vi "REPORT.Rate scan ADD.vi"(9 "Vasic":i32, 10 "Config Test IN":T1={"Config HW"={"VISA Rigol DP832"="USB0::0x1AB1::0x0E11::DP8C191500901::INSTR", "Config Rigol DP832"=[{"Channel"=0, "V Limit"=5.5, "I Limit"=0.5, "V Out"=5.0}, {"Channel"=1, "V Limit"=5.5, "I Limit"=0.8, "V Out"=5.0}, {"Channel"=2, "V Limit"=5.5, "I Limit"=0.2, "V Out"=0.0}], "CTA Test#"="CTA013 A", "FT_Handle"=432921256, "Espera acceso FT"=10, "VISA Tek MDO3104"="Rigol_DP832", "VISA Key 81160A"="Rigol_DP832"}, "Config Test"=[{"Vasic"=2.8, "Global Reset"=FALSE, "Test Register?"=FALSE, "Test ADC?"=FALSE, "Test ADC"={"Repeats ADC"=100, "Max Desviation"=0.1}, "Limits ADC"={"Low"=[1.9, 1.3, 0.65, 0.0, 1.6, 1.4, 1.4, 0.9, 2.1, 0.85, 1.9], "High"=[2.1, 1.5, 0.85, 0.1, 1.4, 1.2, 1.2, 0.7, 1.9, 0.65, 1.7]}, "Test Max PN Min NP?"=FALSE, "Limits Max PN Min NP"={"Max P Upper"=2.177000045776367, "Min P Upper"=1.474, "Max N Upper"=1.475, "Min N Upper"=0.818, "Max P Lower"=1.888, "Min P Lower "=1.321, "Max N Lower"=1.322, "Min N Lower"=0.73}, "Test Rate Scan?"=FALSE, "Vin Rate Scan"=[], "Limits Rate Scan"={"High"=[0.15, 0.242, 0.331, 0.425, 0.512, 0.6, 0.688, 0.774, 0.847, 0.91], "Low"=[0.021, 0.11, 0.189, 0.27, 0.347, 0.421, 0.487, 0.551, 0.601, 0.635]}, "Test Rate Scan Adders?"=FALSE, "Vin Rate Adders"=[], "Limits Rate Scan adders"={"High"=[], "Low"=[]}, "Test offset analog?"=FALSE, "Lim Offset Analog"={"Max Analog"=0.05, "Min Analog"=-0.05}, "Test offset digital?"=FALSE, "Lim offset Dig"={"Max Dig"=0.05}, "Vasic real f.a."=2.8, "IBIAS"=FALSE, "VALUE IBIAS"=63}, {"Vasic"=2.8, "Global Reset"=FALSE, "Test Register?"=FALSE, "Test ADC?"=FALSE, "Test ADC"={"Repeats ADC"=100, "Max Desviation"=0.1}, "Limits ADC"={"Low"=[1.9, 1.3, 0.65, 0.0, 1.6, 1.4, 1.4, 0.9, 2.1, 0.85, 1.9], "High"=[2.1, 1.5, 0.85, 0.1, 1.4, 1.2, 1.2, 0.7, 1.9, 0.65, 1.7]}, "Test Max PN Min NP?"=FALSE, "Limits Max PN Min NP"={"Max P Upper"=2.177000045776367, "Min P Upper"=1.474, "Max N Upper"=1.475, "Min N Upper"=0.818, "Max P Lower"=1.888, "Min P Lower "=1.321, "Max N Lower"=1.322, "Min N Lower"=0.73}, "Test Rate Scan?"=FALSE, "Vin Rate Scan"=[], "Limits Rate Scan"={"High"=[0.15, 0.242, 0.331, 0.425, 0.512, 0.6, 0.688, 0.774, 0.847, 0.91], "Low"=[0.021, 0.11, 0.189, 0.27, 0.347, 0.421, 0.487, 0.551, 0.601, 0.635]}, "Test Rate Scan Adders?"=FALSE, "Vin Rate Adders"=[], "Limits Rate Scan adders"={"High"=[], "Low"=[]}, "Test offset analog?"=FALSE, "Lim Offset Analog"={"Max Analog"=0.05, "Min Analog"=-0.05}, "Test offset digital?"=FALSE, "Lim offset Dig"={"Max Dig"=0.05}, "Vasic real f.a."=2.8, "IBIAS"=FALSE, "VALUE IBIAS"=63}, {"Vasic"=2.8, "Global Reset"=FALSE, "Test Register?"=FALSE, "Test ADC?"=FALSE, "Test ADC"={"Repeats ADC"=100, "Max Desviation"=0.1}, "Limits ADC"={"Low"=[1.9, 1.3, 0.65, 0.0, 1.6, 1.4, 1.4, 0.9, 2.1, 0.85, 1.9], "High"=[2.1, 1.5, 0.85, 0.1, 1.4, 1.2, 1.2, 0.7, 1.9, 0.65, 1.7]}, "Test Max PN Min NP?"=FALSE, "Limits Max PN Min NP"={"Max P Upper"=2.177000045776367, "Min P Upper"=1.474, "Max N Upper"=1.475, "Min N Upper"=0.818, "Max P Lower"=1.888, "Min P Lower "=1.321, "Max N Lower"=1.322, "Min N Lower"=0.73}, "Test Rate Scan?"=FALSE, "Vin Rate Scan"=[], "Limits Rate Scan"={"High"=[0.15, 0.242, 0.331, 0.425, 0.512, 0.6, 0.688, 0.774, 0.847, 0.91], "Low"=[0.021, 0.11, 0.189, 0.27, 0.347, 0.421, 0.487, 0.551, 0.601, 0.635]}, "Test Rate Scan Adders?"=FALSE, "Vin Rate Adders"=[], "Limits Rate Scan adders"={"High"=[], "Low"=[]}, "Test offset analog?"=FALSE, "Lim Offset Analog"={"Max Analog"=0.05, "Min Analog"=-0.05}, "Test offset digital?"=FALSE, "Lim offset Dig"={"Max Dig"=0.05}, "Vasic real f.a."=2.8, "IBIAS"=FALSE, "VALUE IBIAS"=63}, {"Vasic"=2.8, "Global Reset"=FALSE, "Test Register?"=FALSE, "Test ADC?"=FALSE, "Test ADC"={"Repeats ADC"=100, "Max Desviation"=0.1}, "Limits ADC"={"Low"=[1.9, 1.3, 0.65, 0.0, 1.6, 1.4, 1.4, 0.9, 2.1, 0.85, 1.9], "High"=[2.1, 1.5, 0.85, 0.1, 1.4, 1.2, 1.2, 0.7, 1.9, 0.65, 1.7]}, "Test Max PN Min NP?"=FALSE, "Limits Max PN Min NP"={"Max P Upper"=2.177000045776367, "Min P Upper"=1.474, "Max N Upper"=1.475, "Min N Upper"=0.818, "Max P Lower"=1.888, "Min P Lower "=1.321, "Max N Lower"=1.322, "Min N Lower"=0.73}, "Test Rate Scan?"=FALSE, "Vin Rate Scan"=[], "Limits Rate Scan"={"High"=[0.15, 0.242, 0.331, 0.425, 0.512, 0.6, 0.688, 0.774, 0.847, 0.91], "Low"=[0.021, 0.11, 0.189, 0.27, 0.347, 0.421, 0.487, 0.551, 0.601, 0.635]}, "Test Rate Scan Adders?"=FALSE, "Vin Rate Adders"=[], "Limits Rate Scan adders"={"High"=[], "Low"=[]}, "Test offset analog?"=FALSE, "Lim Offset Analog"={"Max Analog"=0.05, "Min Analog"=-0.05}, "Test offset digital?"=FALSE, "Lim offset Dig"={"Max Dig"=0.05}, "Vasic real f.a."=2.8, "IBIAS"=FALSE, "VALUE IBIAS"=63}], "Result"=[{"Vasic Volt"=0, "Test Registros"={"Default Register OK"=TRUE, "Pattern Default"=[6826, 18761, 18761, 18761, 30576, 383, 13312], "Read Default"=[6826, 18761, 18761, 18761, 30576, 383, 13312], "W/R Register OK"=TRUE, "Pattern W/R"=[58709, 46774, 46774, 46774, 34959, 65152, 52223], "Read W/R"=[58709, 46774, 46774, 46774, 34959, 65152, 52223]}, "Test Dacs"={"Desviacion OK"=TRUE, "Means"=[1.9590537240537238, 1.3874725274725273, 0.7671367521367521, 0.020757020757020753, 1.5494139194139194, 1.303919413919414, 1.2742918192918191, 1.2090720390720389, 0.7778327228327229, 2.0368192918192918, 1.8345909645909646], "Deviations"=[0.00042735042735042583, 0.0003965050749137904, 0.00033891407793921574, 3.486925384749193e-18, 0.000366300366300365, 0.0009361009361009328, 0.0010387212621211883, 0.00037241598701881083, 0.0002311318008058711, 0.00043985325898711266, 0.00036630036630038717], "Desviations OK"=[], "Means OK"=[], "Graph Histogram"=[]}, "Test Max-Min PN"={"Max P Mini N OK"=TRUE, "PTHT Max P Min N"=[1.956043956043956, 1.9566544566544566, 1.9566544566544566, 2.034188034188034, 2.0354090354090353, 2.0347985347985347], "PTHT Max P Min N OK"=[TRUE, TRUE, TRUE, TRUE, TRUE, TRUE], "NTHT Max P Min N"=[0.7673992673992674, 0.7673992673992674, 0.7680097680097681, 0.778998778998779, 0.7796092796092796, 0.7796092796092796], "NTHT Max P Min N OK"=[TRUE, TRUE, TRUE, TRUE, TRUE, TRUE], "Min P Max N OK"=TRUE, "PTHT Max N Min P"=[1.387057387057387, 1.387057387057387, 1.387057387057387, 1.4059829059829059, 1.4078144078144077, 1.407203907203907], "PTHT Max N Min P OK"=[TRUE, TRUE, TRUE, TRUE, TRUE, TRUE], "NTHT Max N Min P"=[1.3858363858363858, 1.3846153846153846, 1.3852258852258852, 1.404151404151404, 1.4047619047619047, 1.404151404151404], "NTHT Max N Min P OK"=[TRUE, TRUE, TRUE, TRUE, TRUE, TRUE], "Ref"=[{"DAC THx"=0}, {"DAC THx"=1}, {"DAC THx"=2}, {"DAC THx"=3}, {"DAC THx"=4}, {"DAC THx"=5}]}, "Test Rate Scan"={"Rate Scan OK"=FALSE, "DAC TH0,TH1,TH2"=[], "Volt HLTH"=[], "Rate HLTH OK"=[], "DAC TH3,TH4,TH5"=[], "Volt LLTH"=[], "Rate LLTH 2 OK"=[], "Scaler 0"=[], "Ref"=[], "OFFSET HLTH"=[], "OFFSET LLTH"=[], "Real Voltage"=[]}, "Test Rate Scan adders"={"Rate Scan Adders OK"=FALSE, "DAC TH0,TH1,TH2"=[[[142, 132, 122], [146, 136, 124], [146, 136, 126], [206, 196, 184], [210, 202, 188], [210, 198, 186], [270, 260, 246], [270, 262, 248], [268, 258, 244]], [[248, 238, 222], [250, 242, 226], [250, 242, 228], [358, 348, 330], [360, 352, 334], [358, 350, 334], [460, 452, 434], [462, 454, 438], [458, 450, 434]]], "Volt HLTH"=[[[0.16544566544566552, 0.1562881562881564, 0.14285714285714302], [0.16971916971916978, 0.16117216117216127, 0.14713064713064727], [0.16971916971916978, 0.16117216117216127, 0.14774114774114788], [0.23992673992673996, 0.23015873015873023, 0.21611721611721624], [0.24420024420024422, 0.2362637362637363, 0.2210012210012211], [0.24420024420024422, 0.23137973137973145, 0.21733821733821745], [0.313797313797314, 0.30463980463980467, 0.286935286935287], [0.313797313797314, 0.3058608058608059, 0.2905982905982907], [0.3125763125763128, 0.300976800976801, 0.2851037851037852]], [[0.28937728937728946, 0.2771672771672773, 0.2588522588522588], [0.2905982905982907, 0.28205128205128216, 0.2637362637362637], [0.2905982905982907, 0.28205128205128216, 0.26678876678876673], [0.4157509157509156, 0.4059829059829059, 0.384004884004884], [0.41941391941391926, 0.41086691086691074, 0.38888888888888884], [0.4157509157509156, 0.4072039072039071, 0.38827838827838823], [0.5354090354090353, 0.5268620268620268, 0.5048840048840049], [0.5366300366300365, 0.5274725274725274, 0.5091575091575091], [0.5317460317460316, 0.5225885225885225, 0.5042735042735043]]], "Add HLTH OK"=[], "DAC TH3,TH4,TH5"=[], "Volt LLTH"=[[[134.0, 122.0, 114.0], [136.0, 126.0, 118.0], [136.0, 126.0, 118.0], [192.0, 182.0, 174.0], [194.0, 186.0, 178.0], [194.0, 186.0, 176.0], [250.0, 242.0, 234.0], [254.0, 244.0, 234.0], [250.0, 240.0, 230.0]], [[230.0, 220.0, 212.0], [234.0, 224.0, 214.0], [234.0, 224.0, 214.0], [338.0, 326.0, 316.0], [338.0, 330.0, 320.0], [338.0, 328.0, 318.0], [436.0, 424.0, 416.0], [438.0, 426.0, 416.0], [434.0, 422.0, 414.0]]], "Add LLTH 2 OK"=[], "Scaler 0"=[[[1, 1, 1], [1, 1, 1], [1, 1, 1], [0, 0, 0], [0, 0, 0], [0, 0, 0], [0, 0, 0], [0, 0, 0], [0, 0, 0]], [[1, 1, 1], [1, 1, 1], [1, 1, 1], [0, 1, 1], [0, 1, 1], [0, 1, 1], [0, 0, 0], [0, 0, 0], [0, 0, 0]]], "Ref"=[], "OFFSET HLTH"=[], "OFFSET LLTH"=[], "Real Voltage"=[]}, "Test Offset Analog"={"Offset Analog OK"=FALSE, "V ADDOUT"=[], "Offset OK"=[], "Ref"=[]}, "Test Offset Digital"={"Offset Digital OK"=FALSE, "SCALER 1 START"=[], "SCALER 1 STOP"=[], "THX START"=[], "THX STOP"=[], "VHLTH START"=[], "VHLTH STOP"=[], "Index 1 Start"=[], "index 1 Stop"=[], "SCALER 2 START"=[], "SCALER 2 STOP"=[], "THX+3 START"=[], "THX+3 STOP"=[], "VLLTH START"=[], "VLLTH STOP"=[], "Index 2 Start"=[], "index 2 Stop"=[], "Dig HLTH OK"=[], "Dig LLTH 2 OK"=[], "Ref"=[]}, "info hardware"={"Iout V1"=0.0, "Iout V2"=0.0, "Iout V3"=0.0, "Vout V1"=0.0, "Vout V2"=0.0, "Vout V3"=0.0, "Temp"=0.0}, "Test Offset Analog add"={"Offset Analog add OK"=FALSE, "V ADDOUT add"=[], "Offset add OK"=[], "Ref add"=[]}, "info temp"={"T Asic Registers"=0.0, "T Board Test. ADC"=0.0, "T Asic Max Min N P"=0.0, "T Adc count"=0.0, "T Asic Digital Offset"=0.0, "T Asic Analog Offset"=0.0, "T Asic Analog add"=0.0, "T Asic Rate Scan"=0.0, "T Asic Rate Scan Adders"=0.0, "T Final"=0.0}}, {"Vasic Volt"=0, "Test Registros"={"Default Register OK"=TRUE, "Pattern Default"=[6826, 18761, 18761, 18761, 30576, 383, 13312], "Read Default"=[6826, 18761, 18761, 18761, 30576, 383, 13312], "W/R Register OK"=TRUE, "Pattern W/R"=[58709, 46774, 46774, 46774, 34959, 65152, 52223], "Read W/R"=[58709, 46774, 46774, 46774, 34959, 65152, 52223]}, "Test Dacs"={"Desviacion OK"=TRUE, "Means"=[1.9590537240537238, 1.3874725274725273, 0.7671367521367521, 0.020757020757020753, 1.5494139194139194, 1.303919413919414, 1.2742918192918191, 1.2090720390720389, 0.7778327228327229, 2.0368192918192918, 1.8345909645909646], "Deviations"=[0.00042735042735042583, 0.0003965050749137904, 0.00033891407793921574, 3.486925384749193e-18, 0.000366300366300365, 0.0009361009361009328, 0.0010387212621211883, 0.00037241598701881083, 0.0002311318008058711, 0.00043985325898711266, 0.00036630036630038717], "Desviations OK"=[], "Means OK"=[], "Graph Histogram"=[]}, "Test Max-Min PN"={"Max P Mini N OK"=TRUE, "PTHT Max P Min N"=[1.956043956043956, 1.9566544566544566, 1.9566544566544566, 2.034188034188034, 2.0354090354090353, 2.0347985347985347], "PTHT Max P Min N OK"=[TRUE, TRUE, TRUE, TRUE, TRUE, TRUE], "NTHT Max P Min N"=[0.7673992673992674, 0.7673992673992674, 0.7680097680097681, 0.778998778998779, 0.7796092796092796, 0.7796092796092796], "NTHT Max P Min N OK"=[TRUE, TRUE, TRUE, TRUE, TRUE, TRUE], "Min P Max N OK"=TRUE, "PTHT Max N Min P"=[1.387057387057387, 1.387057387057387, 1.387057387057387, 1.4059829059829059, 1.4078144078144077, 1.407203907203907], "PTHT Max N Min P OK"=[TRUE, TRUE, TRUE, TRUE, TRUE, TRUE], "NTHT Max N Min P"=[1.3858363858363858, 1.3846153846153846, 1.3852258852258852, 1.404151404151404, 1.4047619047619047, 1.404151404151404], "NTHT Max N Min P OK"=[TRUE, TRUE, TRUE, TRUE, TRUE, TRUE], "Ref"=[{"DAC THx"=0}, {"DAC THx"=1}, {"DAC THx"=2}, {"DAC THx"=3}, {"DAC THx"=4}, {"DAC THx"=5}]}, "Test Rate Scan"={"Rate Scan OK"=FALSE, "DAC TH0,TH1,TH2"=[], "Volt HLTH"=[], "Rate HLTH OK"=[], "DAC TH3,TH4,TH5"=[], "Volt LLTH"=[], "Rate LLTH 2 OK"=[], "Scaler 0"=[], "Ref"=[], "OFFSET HLTH"=[], "OFFSET LLTH"=[], "Real Voltage"=[]}, "Test Rate Scan adders"={"Rate Scan Adders OK"=FALSE, "DAC TH0,TH1,TH2"=[], "Volt HLTH"=[], "Add HLTH OK"=[], "DAC TH3,TH4,TH5"=[], "Volt LLTH"=[], "Add LLTH 2 OK"=[], "Scaler 0"=[], "Ref"=[], "OFFSET HLTH"=[], "OFFSET LLTH"=[], "Real Voltage"=[]}, "Test Offset Analog"={"Offset Analog OK"=FALSE, "V ADDOUT"=[], "Offset OK"=[], "Ref"=[]}, "Test Offset Digital"={"Offset Digital OK"=FALSE, "SCALER 1 START"=[], "SCALER 1 STOP"=[], "THX START"=[], "THX STOP"=[], "VHLTH START"=[], "VHLTH STOP"=[], "Index 1 Start"=[], "index 1 Stop"=[], "SCALER 2 START"=[], "SCALER 2 STOP"=[], "THX+3 START"=[], "THX+3 STOP"=[], "VLLTH START"=[], "VLLTH STOP"=[], "Index 2 Start"=[], "index 2 Stop"=[], "Dig HLTH OK"=[], "Dig LLTH 2 OK"=[], "Ref"=[]}, "info hardware"={"Iout V1"=0.0, "Iout V2"=0.0, "Iout V3"=0.0, "Vout V1"=0.0, "Vout V2"=0.0, "Vout V3"=0.0, "Temp"=0.0}, "Test Offset Analog add"={"Offset Analog add OK"=FALSE, "V ADDOUT add"=[], "Offset add OK"=[], "Ref add"=[]}, "info temp"={"T Asic Registers"=0.0, "T Board Test. ADC"=0.0, "T Asic Max Min N P"=0.0, "T Adc count"=0.0, "T Asic Digital Offset"=0.0, "T Asic Analog Offset"=0.0, "T Asic Analog add"=0.0, "T Asic Rate Scan"=0.0, "T Asic Rate Scan Adders"=0.0, "T Final"=0.0}}, {"Vasic Volt"=0, "Test Registros"={"Default Register OK"=TRUE, "Pattern Default"=[6826, 18761, 18761, 18761, 30576, 383, 13312], "Read Default"=[6826, 18761, 18761, 18761, 30576, 383, 13312], "W/R Register OK"=TRUE, "Pattern W/R"=[58709, 46774, 46774, 46774, 34959, 65152, 52223], "Read W/R"=[58709, 46774, 46774, 46774, 34959, 65152, 52223]}, "Test Dacs"={"Desviacion OK"=TRUE, "Means"=[1.9590537240537238, 1.3874725274725273, 0.7671367521367521, 0.020757020757020753, 1.5494139194139194, 1.303919413919414, 1.2742918192918191, 1.2090720390720389, 0.7778327228327229, 2.0368192918192918, 1.8345909645909646], "Deviations"=[0.00042735042735042583, 0.0003965050749137904, 0.00033891407793921574, 3.486925384749193e-18, 0.000366300366300365, 0.0009361009361009328, 0.0010387212621211883, 0.00037241598701881083, 0.0002311318008058711, 0.00043985325898711266, 0.00036630036630038717], "Desviations OK"=[], "Means OK"=[], "Graph Histogram"=[]}, "Test Max-Min PN"={"Max P Mini N OK"=FALSE, "PTHT Max P Min N"=[], "PTHT Max P Min N OK"=[], "NTHT Max P Min N"=[], "NTHT Max P Min N OK"=[], "Min P Max N OK"=FALSE, "PTHT Max N Min P"=[], "PTHT Max N Min P OK"=[], "NTHT Max N Min P"=[], "NTHT Max N Min P OK"=[], "Ref"=[]}, "Test Rate Scan"={"Rate Scan OK"=FALSE, "DAC TH0,TH1,TH2"=[], "Volt HLTH"=[], "Rate HLTH OK"=[], "DAC TH3,TH4,TH5"=[], "Volt LLTH"=[], "Rate LLTH 2 OK"=[], "Scaler 0"=[], "Ref"=[], "OFFSET HLTH"=[], "OFFSET LLTH"=[], "Real Voltage"=[]}, "Test Rate Scan adders"={"Rate Scan Adders OK"=FALSE, "DAC TH0,TH1,TH2"=[], "Volt HLTH"=[], "Add HLTH OK"=[], "DAC TH3,TH4,TH5"=[], "Volt LLTH"=[], "Add LLTH 2 OK"=[], "Scaler 0"=[], "Ref"=[], "OFFSET HLTH"=[], "OFFSET LLTH"=[], "Real Voltage"=[]}, "Test Offset Analog"={"Offset Analog OK"=FALSE, "V ADDOUT"=[], "Offset OK"=[], "Ref"=[]}, "Test Offset Digital"={"Offset Digital OK"=FALSE, "SCALER 1 START"=[], "SCALER 1 STOP"=[], "THX START"=[], "THX STOP"=[], "VHLTH START"=[], "VHLTH STOP"=[], "Index 1 Start"=[], "index 1 Stop"=[], "SCALER 2 START"=[], "SCALER 2 STOP"=[], "THX+3 START"=[], "THX+3 STOP"=[], "VLLTH START"=[], "VLLTH STOP"=[], "Index 2 Start"=[], "index 2 Stop"=[], "Dig HLTH OK"=[], "Dig LLTH 2 OK"=[], "Ref"=[]}, "info hardware"={"Iout V1"=0.0, "Iout V2"=0.0, "Iout V3"=0.0, "Vout V1"=0.0, "Vout V2"=0.0, "Vout V3"=0.0, "Temp"=0.0}, "Test Offset Analog add"={"Offset Analog add OK"=FALSE, "V ADDOUT add"=[], "Offset add OK"=[], "Ref add"=[]}, "info temp"={"T Asic Registers"=0.0, "T Board Test. ADC"=0.0, "T Asic Max Min N P"=0.0, "T Adc count"=0.0, "T Asic Digital Offset"=0.0, "T Asic Analog Offset"=0.0, "T Asic Analog add"=0.0, "T Asic Rate Scan"=0.0, "T Asic Rate Scan Adders"=0.0, "T Final"=0.0}}, {"Vasic Volt"=0, "Test Registros"={"Default Register OK"=TRUE, "Pattern Default"=[6826, 18761, 18761, 18761, 30576, 383, 13312], "Read Default"=[6826, 18761, 18761, 18761, 30576, 383, 13312], "W/R Register OK"=TRUE, "Pattern W/R"=[58709, 46774, 46774, 46774, 34959, 65152, 52223], "Read W/R"=[58709, 46774, 46774, 46774, 34959, 65152, 52223]}, "Test Dacs"={"Desviacion OK"=FALSE, "Means"=[], "Deviations"=[], "Desviations OK"=[], "Means OK"=[], "Graph Histogram"=[]}, "Test Max-Min PN"={"Max P Mini N OK"=FALSE, "PTHT Max P Min N"=[], "PTHT Max P Min N OK"=[], "NTHT Max P Min N"=[], "NTHT Max P Min N OK"=[], "Min P Max N OK"=FALSE, "PTHT Max N Min P"=[], "PTHT Max N Min P OK"=[], "NTHT Max N Min P"=[], "NTHT Max N Min P OK"=[], "Ref"=[]}, "Test Rate Scan"={"Rate Scan OK"=FALSE, "DAC TH0,TH1,TH2"=[], "Volt HLTH"=[], "Rate HLTH OK"=[], "DAC TH3,TH4,TH5"=[], "Volt LLTH"=[], "Rate LLTH 2 OK"=[], "Scaler 0"=[], "Ref"=[], "OFFSET HLTH"=[], "OFFSET LLTH"=[], "Real Voltage"=[]}, "Test Rate Scan adders"={"Rate Scan Adders OK"=FALSE, "DAC TH0,TH1,TH2"=[], "Volt HLTH"=[], "Add HLTH OK"=[], "DAC TH3,TH4,TH5"=[], "Volt LLTH"=[], "Add LLTH 2 OK"=[], "Scaler 0"=[], "Ref"=[], "OFFSET HLTH"=[], "OFFSET LLTH"=[], "Real Voltage"=[]}, "Test Offset Analog"={"Offset Analog OK"=FALSE, "V ADDOUT"=[], "Offset OK"=[], "Ref"=[]}, "Test Offset Digital"={"Offset Digital OK"=FALSE, "SCALER 1 START"=[], "SCALER 1 STOP"=[], "THX START"=[], "THX STOP"=[], "VHLTH START"=[], "VHLTH STOP"=[], "Index 1 Start"=[], "index 1 Stop"=[], "SCALER 2 START"=[], "SCALER 2 STOP"=[], "THX+3 START"=[], "THX+3 STOP"=[], "VLLTH START"=[], "VLLTH STOP"=[], "Index 2 Start"=[], "index 2 Stop"=[], "Dig HLTH OK"=[], "Dig LLTH 2 OK"=[], "Ref"=[]}, "info hardware"={"Iout V1"=0.0, "Iout V2"=0.0, "Iout V3"=0.0, "Vout V1"=0.0, "Vout V2"=0.0, "Vout V3"=0.0, "Temp"=0.0}, "Test Offset Analog add"={"Offset Analog add OK"=FALSE, "V ADDOUT add"=[], "Offset add OK"=[], "Ref add"=[]}, "info temp"={"T Asic Registers"=0.0, "T Board Test. ADC"=0.0, "T Asic Max Min N P"=0.0, "T Adc count"=0.0, "T Asic Digital Offset"=0.0, "T Asic Analog Offset"=0.0, "T Asic Analog add"=0.0, "T Asic Rate Scan"=0.0, "T Asic Rate Scan Adders"=0.0, "T Final"=0.0}}], "Execucion Test"={"Vasic Actual"=0}, "Config VGA"={"Theoretical Voltage"=[0.1, 0.2, 0.3, 0.4, 0.5, 0.6, 0.7, 0.8, 0.9, 1.0], "Real Voltage"=[0.10285, 0.20714, 0.29957, 0.40485, 0.49571, 0.60685, 0.69771, 0.80114, 0.89714, 0.99885], "Pulse Width"=57344, "Frecuency Pulse"=1000000.0, "VGA Gain"=[9, 16, 24, 34, 43, 52, 61, 72, 81, 93]}, "Test Info"={"Asic"="", "Operator"="", "Place"="", "Time start"=timestamp(0 s since 1904-01-01), "Time stop"=timestamp(0 s since 1904-01-01)}, "Info machine"={"SO"="", "SO Name"="", "SO Ver"="", "SO Build"="", "CPU"="", "APP"="", "APP YEAR"="", "APP ver"="", "APP User"="", "APP Serail"="", "MAC"=[], "PC NAME"=[], "PC IP"=[], "BIOS MANU"="", "BIOS NAME"="", "BIOS SERIAL"="", "BOARD MANU"="", "BOARD NAME"="", "BOARD SERIAL"="", "Driver Version"="", "Library Version"="", "FPGA Ver"=0, "ID CTA board"=0, "LAST BOOT"="", "LABVIEW Ver"=0}, "Partial Report"="", "CONFIG GEN"=[]} {"CONFIG GEN"."Vasic Theorical" min=1.0 max=1000000.0 step=1.0 format="%#_6pV"; "CONFIG GEN"."Frequency" min=0.001 max=333000000.0 step=1000.0 format="%#_6pHz"; "CONFIG GEN"."Leading Edge Time" min=1e-09 max=1.0 step=1e-10 format="%#_6ps"; "CONFIG GEN"."Trailing Edge Time" min=1e-09 max=1.0 step=1e-10 format="%#_6ps"; "CONFIG GEN"."Delay" min=0.0 max=1.0 step=1e-12 format="%#_6ps"; "CONFIG GEN"."Trigger Level Sync" items=["ECL", "TTL"]; "CONFIG GEN"."Trigger Sync Out" items=["AB"=3, "B"=2, "A"=1, "None"=0]; "CONFIG GEN"."Load" min=1.0 max=1000000.0 step=1.0 format="%#_6p"; "CONFIG GEN"."DC Offset" min=-10.0 max=10.0 step=0.1 format="%#_6pV"; "CONFIG GEN"."Amplitude" min=0.05 max=5.0 step=0.001 format="%#_6pV"; "CONFIG GEN"."Width Time" min=1.5e-09 max=1.0 step=1e-10 format="%#_6ps"; "CONFIG GEN"."Channel" items=["Channel1"=1, "Channel2"=2]; "Config VGA"."Theoretical Voltage" format="%1.4f"; "Config VGA"."VGA Gain" format="%02x"; "Config VGA"."Frecuency Pulse" format="%0_2p"; "Config VGA"."Pulse Width" format="%04x"; "Config VGA"."Real Voltage" format="%1.5f"; "Config Test"."VALUE IBIAS" max=63 step=1; "Config Test"."Vasic real f.a." min=2.8 max=3.8 step=0.01 format="%.2g"; "Config Test"."Limits Rate Scan adders"."Low" format="%1.3f"; "Config Test"."Limits Rate Scan adders"."High" format="%1.3f"; "Config Test"."Limits ADC"."High" format="%1.4f"; "Config Test"."Limits ADC"."Low" format="%1.3f"; "Config Test"."Lim offset Dig"."Max Dig" format="%.3g"; "Config Test"."Lim Offset Analog"."Min Analog" format="%.3g"; "Config Test"."Lim Offset Analog"."Max Analog" format="%.3g"; "Config Test"."Limits Rate Scan"."Low" format="%1.4f"; "Config Test"."Limits Rate Scan"."High" format="%1.3f"; "Config Test"."Limits Max PN Min NP"."Min P Upper" format="%.3g"; "Config Test"."Limits Max PN Min NP"."Min P Lower" format="%.3g"; "Config Test"."Limits Max PN Min NP"."Max N Lower" format="%.3g"; "Config Test"."Limits Max PN Min NP"."Max N Upper" format="%.3g"; "Config Test"."Limits Max PN Min NP"."Min N Lower" format="%.3g"; "Config Test"."Limits Max PN Min NP"."Min N Upper" format="%.3g"; "Config Test"."Limits Max PN Min NP"."Max P Upper" format="%.3g"; "Config Test"."Limits Max PN Min NP"."Max P Lower" format="%.3g"; "Config Test"."Vasic" min=2.8 max=3.8 step=0.01 format="%.2g"; "Config HW"."Config Rigol DP832"."Channel" items=["+30V Channel 1", "+30V Channel 2", "+5V Channel 3"]; "Config HW"."Config Rigol DP832"."V Limit" format="%.1g"; "Config HW"."Config Rigol DP832"."I Limit" format="%.1g"; "Config HW"."Config Rigol DP832"."V Out" format="%.1g"; "Result"."Test Registros"."Read W/R" format="%04x"; "Result"."Test Registros"."Pattern W/R" format="%04x"; "Result"."Test Registros"."Read Default" format="%04x"; "Result"."Test Registros"."Pattern Default" format="%04x"}, 11 "Text In":string) -> (3 "Text Out":string)   [LabVIEW 2019]
uses:
  Test.ctl
  TEST.TEST CONFIG HW.ctl
  Rigol DP832/DP832_Control Channels.ctl
  TEST.TEST CONFIG TEST MATRIZ.ctl
  TEST.TEST CONFIG TEST.ctl
  TEST.TEST RESULT.ctl
  test_result fvasic.ctl
  TEST.TEST EXECUTION TEST.ctl
  TEST.TEST CONFIG VGA.ctl
  TEST.TEST TEST INFO.ctl
  TEST.TEST INFO PC.ctl
  GenPulse_configurar.ctl
panel:
  # "Modo 2\nModo 3\nModo 4\nModo 2\nModo 3\nModo 4"
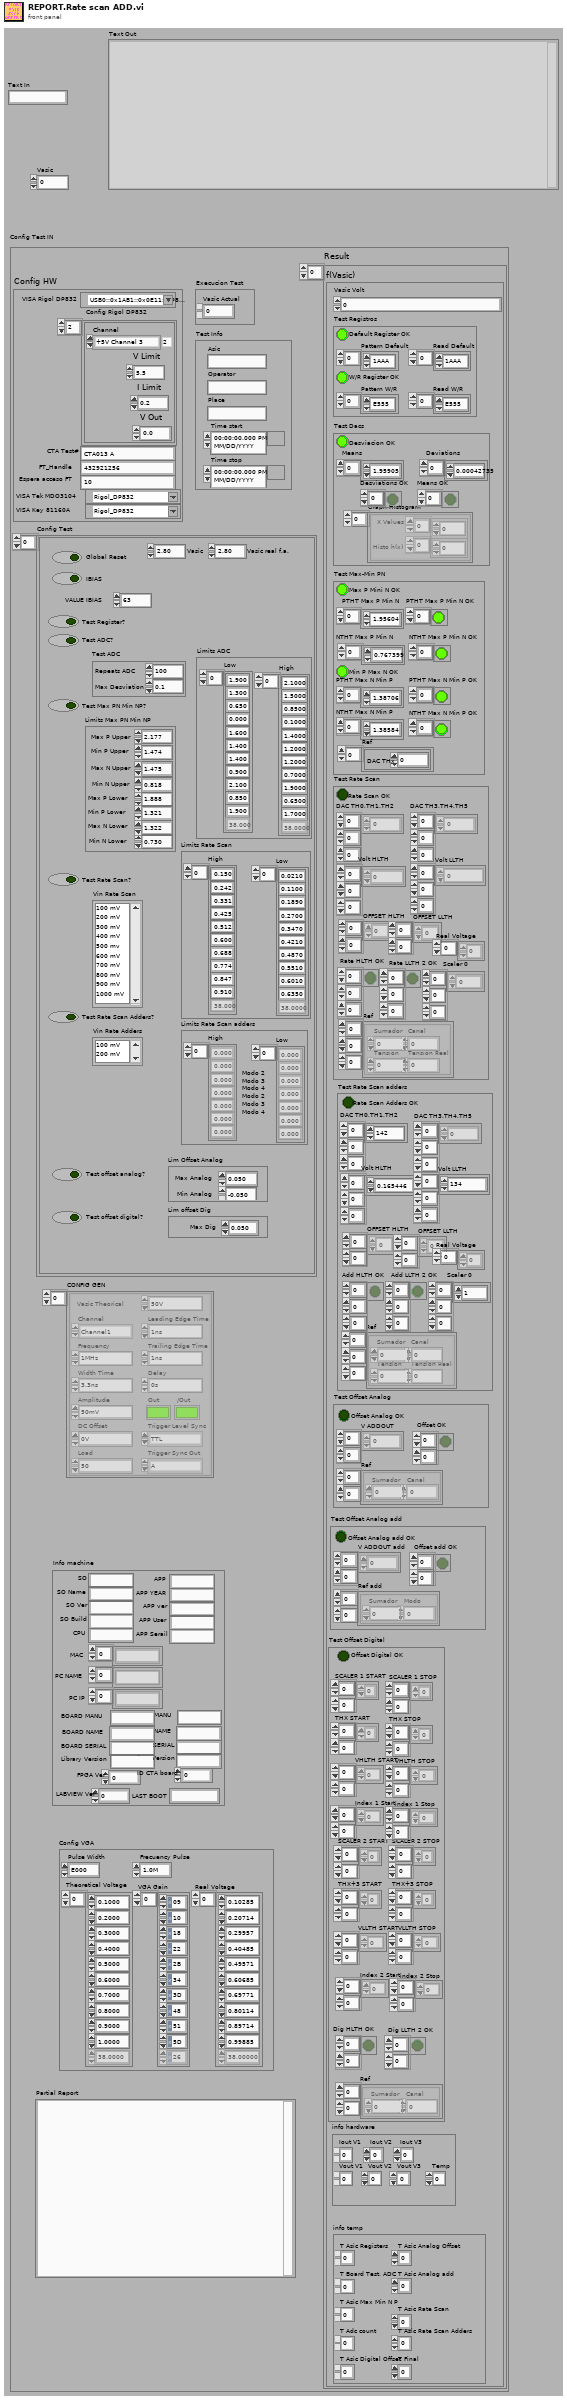
[diagram p1: front panel]
types:
  T1 = typedef "Test.ctl" = cluster{"Config HW":T2, "Config Test":T4, "Result":T6, "Execucion Test":T8, "Config VGA":T9, "Test Info":T10, "Info machine":T11, "Partial Report":string, "CONFIG GEN":T12[]}
  T2 = typedef "TEST.TEST CONFIG HW.ctl" = cluster{"VISA Rigol DP832":refnum<visa-resource-name>, "Config Rigol DP832":cluster{"Channel":T3, "V Limit":dbl, "I Limit":dbl, "V Out":dbl}[], "CTA Test#":string, "FT_Handle":u32, "Espera acceso FT":u32, "VISA Tek MDO3104":refnum<visa-resource-name>, "VISA Key 81160A":refnum<visa-resource-name>}
  T3 = typedef "DP832_Control Channels.ctl" = i32
  T4 = typedef "TEST.TEST CONFIG TEST MATRIZ.ctl" = T5[]
  T5 = typedef "TEST.TEST CONFIG TEST.ctl" = cluster{"Vasic":dbl, "Global Reset":bool, "Test Register?":bool, "Test ADC?":bool, "Test ADC":cluster{"Repeats ADC":i32, "Max Desviation":dbl}, "Limits ADC":cluster{"Low":dbl[], "High":dbl[]}, "Test Max PN Min NP?":bool, "Limits Max PN Min NP":cluster{"Max P Upper":dbl, "Min P Upper":dbl, "Max N Upper":dbl, "Min N Upper":dbl, "Max P Lower":dbl, "Min P Lower ":dbl, "Max N Lower":dbl, "Min N Lower":dbl}, "Test Rate Scan?":bool, "Vin Rate Scan":i32[], "Limits Rate Scan":cluster{"High":dbl[], "Low":dbl[]}, "Test Rate Scan Adders?":bool, "Vin Rate Adders":i32[], "Limits Rate Scan adders":cluster{"High":dbl[], "Low":dbl[]}, "Test offset analog?":bool, "Lim Offset Analog":cluster{"Max Analog":dbl, "Min Analog":dbl}, "Test offset digital?":bool, "Lim offset Dig":cluster{"Max Dig":dbl}, "Vasic real f.a.":dbl, "IBIAS":bool, "VALUE IBIAS":u8}
  T6 = typedef "TEST.TEST RESULT.ctl" = T7[]
  T7 = typedef "test_result fvasic.ctl" = cluster{"Vasic Volt":i32, "Test Registros":cluster{"Default Register OK":bool, "Pattern Default":u16[], "Read Default":u16[], "W/R Register OK":bool, "Pattern W/R":u16[], "Read W/R":u16[]}, "Test Dacs":cluster{"Desviacion OK":bool, "Means":dbl[], "Deviations":dbl[], "Desviations OK":bool[], "Means OK":bool[], "Graph Histogram":cluster{"X Values":dbl[], "Histo h(x)":i32[]}[]}, "Test Max-Min PN":cluster{"Max P Mini N OK":bool, "PTHT Max P Min N":dbl[], "PTHT Max P Min N OK":bool[], "NTHT Max P Min N":dbl[], "NTHT Max P Min N OK":bool[], "Min P Max N OK":bool, "PTHT Max N Min P":dbl[], "PTHT Max N Min P OK":bool[], "NTHT Max N Min P":dbl[], "NTHT Max N Min P OK":bool[], "Ref":cluster{"DAC THx":u8}[]}, "Test Rate Scan":cluster{"Rate Scan OK":bool, "DAC TH0,TH1,TH2":u16[][][], "Volt HLTH":dbl[][][], "Rate HLTH OK":bool[][][], "DAC TH3,TH4,TH5":u16[][][], "Volt LLTH":dbl[][][], "Rate LLTH 2 OK":bool[][][], "Scaler 0":u16[][][], "Ref":cluster{"Sumador":u8, "Canal":u8, "Tension":u8, "Tension Real":dbl}[][][], "OFFSET HLTH":dbl[][], "OFFSET LLTH":dbl[][], "Real Voltage":dbl[]}, "Test Rate Scan adders":cluster{"Rate Scan Adders OK":bool, "DAC TH0,TH1,TH2":u16[][][], "Volt HLTH":dbl[][][], "Add HLTH OK":bool[][][], "DAC TH3,TH4,TH5":u16[][][], "Volt LLTH":dbl[][][], "Add LLTH 2 OK":bool[][][], "Scaler 0":u16[][][], "Ref":cluster{"Sumador":u8, "Canal":u8, "Tension":u8, "Tension Real":dbl}[][][], "OFFSET HLTH":dbl[][], "OFFSET LLTH":dbl[][], "Real Voltage":dbl[]}, "Test Offset Analog":cluster{"Offset Analog OK":bool, "V ADDOUT":dbl[][], "Offset OK":bool[][], "Ref":cluster{"Sumador":u8, "Canal":u8}[][]}, "Test Offset Digital":cluster{"Offset Digital OK":bool, "SCALER 1 START":u16[][], "SCALER 1 STOP":u16[][], "THX START":u16[][], "THX STOP":u16[][], "VHLTH START":dbl[][], "VHLTH STOP":dbl[][], "Index 1 Start":i32[][], "index 1 Stop":i32[][], "SCALER 2 START":u16[][], "SCALER 2 STOP":u16[][], "THX+3 START":u16[][], "THX+3 STOP":u16[][], "VLLTH START":dbl[][], "VLLTH STOP":dbl[][], "Index 2 Start":i32[][], "index 2 Stop":i32[][], "Dig HLTH OK":bool[][], "Dig LLTH 2 OK":bool[][], "Ref":cluster{"Sumador":u8, "Canal":u8}[][]}, "info hardware":cluster{"Iout V1":dbl, "Iout V2":dbl, "Iout V3":dbl, "Vout V1":dbl, "Vout V2":dbl, "Vout V3":dbl, "Temp":dbl}, "Test Offset Analog add":cluster{"Offset Analog add OK":bool, "V ADDOUT add":dbl[][], "Offset add OK":bool[][], "Ref add":cluster{"Sumador":u8, "Modo":u8}[][]}, "info temp":cluster{"T Asic Registers":dbl, "T Board Test. ADC":dbl, "T Asic Max Min N P":dbl, "T Adc count":dbl, "T Asic Digital Offset":dbl, "T Asic Analog Offset":dbl, "T Asic Analog add":dbl, "T Asic Rate Scan":dbl, "T Asic Rate Scan Adders":dbl, "T Final":dbl}}
  T8 = typedef "TEST.TEST EXECUTION TEST.ctl" = cluster{"Vasic Actual":i32}
  T9 = typedef "TEST.TEST CONFIG VGA.ctl" = cluster{"Theoretical Voltage":dbl[], "Real Voltage":dbl[], "Pulse Width":u16, "Frecuency Pulse":dbl, "VGA Gain":u8[]}
  T10 = typedef "TEST.TEST TEST INFO.ctl" = cluster{"Asic":string, "Operator":string, "Place":string, "Time start":timestamp, "Time stop":timestamp}
  T11 = typedef "TEST.TEST INFO PC.ctl" = cluster{"SO":string, "SO Name":string, "SO Ver":string, "SO Build":string, "CPU":string, "APP":string, "APP YEAR":string, "APP ver":string, "APP User":string, "APP Serail":string, "MAC":string[], "PC NAME":string[], "PC IP":string[], "BIOS MANU":string, "BIOS NAME":string, "BIOS SERIAL":string, "BOARD MANU":string, "BOARD NAME":string, "BOARD SERIAL":string, "Driver Version":string, "Library Version":string, "FPGA Ver":u8, "ID CTA board":u64, "LAST BOOT":string, "LABVIEW Ver":u32}
  T12 = typedef "GenPulse_configurar.ctl" = cluster{"Channel":u16, "Frequency":dbl, "Width Time":dbl, "Amplitude":dbl, "DC Offset":dbl, "Load":dbl, "Leading Edge Time":dbl, "Trailing Edge Time":dbl, "Delay":dbl, "Out":bool, "/Out":bool, "Trigger Level Sync":u16, "Trigger Sync Out":u16, "Vasic Theorical":dbl}
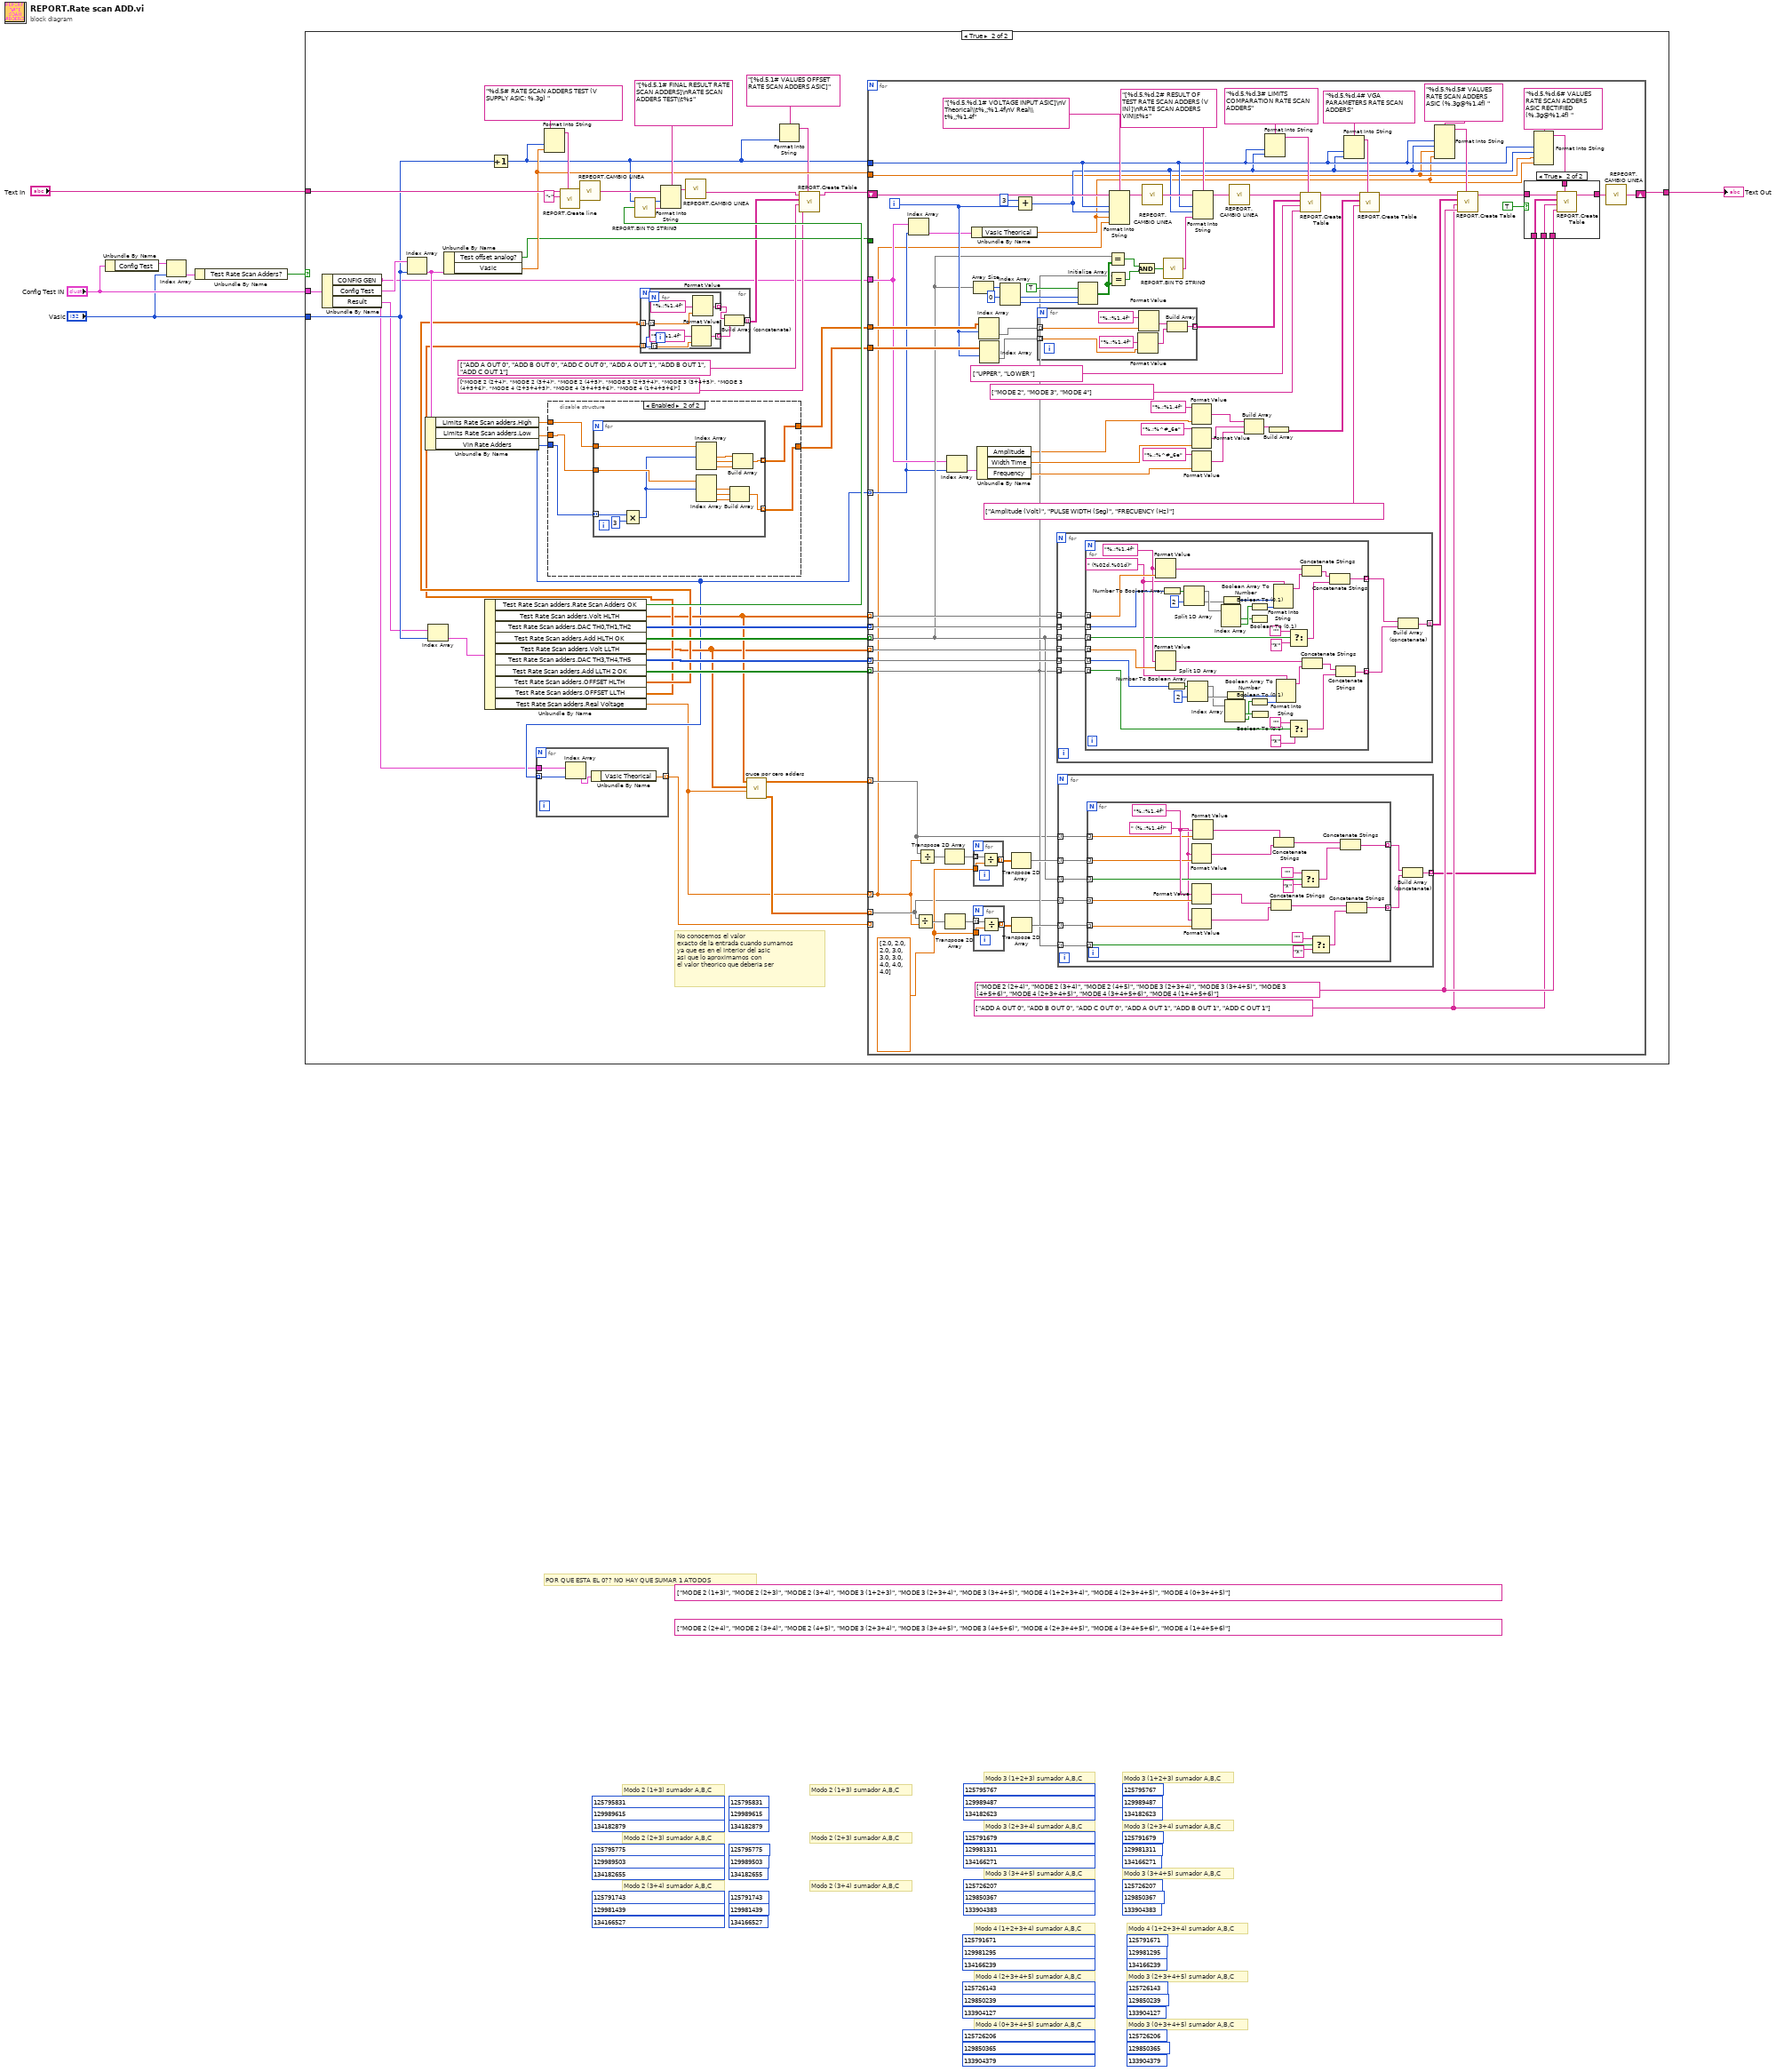
[diagram p0: block diagram]
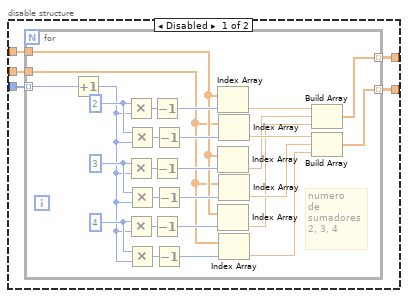
[diagram p3: hidden frame]
diagram:
  (unwired) string[] ["MODE 2 (1+3)", "MODE 2 (2+3)", "MODE 2 (3+4)", "MODE 3 (1+2+3)", "MODE 3 (2+3+4)", "MODE 3 (3+4+5)", "MODE 4 (1+2+3+4)", "MODE 4 (2+3+4+5)", "MODE 4 (0+3+4+5)"] ("Column Headers")
  (unwired) string[] ["MODE 2 (2+4)", "MODE 2 (3+4)", "MODE 2 (4+5)", "MODE 3 (2+3+4)", "MODE 3 (3+4+5)", "MODE 3 (4+5+6)", "MODE 4 (2+3+4+5)", "MODE 4 (3+4+5+6)", "MODE 4 (1+4+5+6)"] ("Column Headers")
  (unwired) u32 134166527 ("Threshold Inicial N")
  (unwired) u32 129981439 ("Threshold Inicial N")
  (unwired) u32 125791743 ("Threshold Inicial N")
  (unwired) u32 134182655 ("Threshold Inicial N")
  (unwired) u32 129989503 ("Threshold Inicial N")
  (unwired) u32 125795775 ("Threshold Inicial N")
  (unwired) u32 134182879 ("Threshold Inicial N")
  (unwired) u32 129989615 ("Threshold Inicial N")
  (unwired) u32 125795831 ("Threshold Inicial N")
  (unwired) u32 134166527 ("Threshold Inicial N")
  (unwired) u32 129981439 ("Threshold Inicial N")
  (unwired) u32 125791743 ("Threshold Inicial N")
  (unwired) u32 134182655 ("Threshold Inicial N")
  (unwired) u32 129989503 ("Threshold Inicial N")
  (unwired) u32 125795775 ("Threshold Inicial N")
  (unwired) u32 134182879 ("Threshold Inicial N")
  (unwired) u32 129989615 ("Threshold Inicial N")
  (unwired) u32 125795831 ("Threshold Inicial N")
  (unwired) u32 133904379 ("Threshold Inicial N")
  (unwired) u32 129850365 ("Threshold Inicial N")
  (unwired) u32 125726206 ("Threshold Inicial N")
  (unwired) u32 133904127 ("Threshold Inicial N")
  (unwired) u32 129850239 ("Threshold Inicial N")
  (unwired) u32 125726143 ("Threshold Inicial N")
  (unwired) u32 134166239 ("Threshold Inicial N")
  (unwired) u32 129981295 ("Threshold Inicial N")
  (unwired) u32 125791671 ("Threshold Inicial N")
  (unwired) u32 133904379 ("Threshold Inicial N")
  (unwired) u32 129850365 ("Threshold Inicial N")
  (unwired) u32 125726206 ("Threshold Inicial N")
  (unwired) u32 133904127 ("Threshold Inicial N")
  (unwired) u32 129850239 ("Threshold Inicial N")
  (unwired) u32 125726143 ("Threshold Inicial N")
  (unwired) u32 134166239 ("Threshold Inicial N")
  (unwired) u32 129981295 ("Threshold Inicial N")
  (unwired) u32 125791671 ("Threshold Inicial N")
  (unwired) u32 133904383 ("Threshold Inicial N")
  (unwired) u32 129850367 ("Threshold Inicial N")
  (unwired) u32 125726207 ("Threshold Inicial N")
  (unwired) u32 134166271 ("Threshold Inicial N")
  (unwired) u32 129981311 ("Threshold Inicial N")
  (unwired) u32 125791679 ("Threshold Inicial N")
  (unwired) u32 134182623 ("Threshold Inicial N")
  (unwired) u32 129989487 ("Threshold Inicial N")
  (unwired) u32 125795767 ("Threshold Inicial N")
  (unwired) u32 133904383 ("Threshold Inicial N")
  (unwired) u32 129850367 ("Threshold Inicial N")
  (unwired) u32 125726207 ("Threshold Inicial N")
  (unwired) u32 134166271 ("Threshold Inicial N")
  (unwired) u32 129981311 ("Threshold Inicial N")
  (unwired) u32 125791679 ("Threshold Inicial N")
  (unwired) u32 134182623 ("Threshold Inicial N")
  (unwired) u32 129989487 ("Threshold Inicial N")
  (unwired) u32 125795767 ("Threshold Inicial N")
  # "POR QUE ESTA EL 0?? NO HAY QUE SUMAR 1 ATODOS"
  # "Modo 2 (3+4) sumador A,B,C"
  # "Modo 2 (2+3) sumador A,B,C"
  # "Modo 2 (1+3) sumador A,B,C"
  # "Modo 2 (3+4) sumador A,B,C"
  # "Modo 2 (2+3) sumador A,B,C"
  # "Modo 2 (1+3) sumador A,B,C"
  # "Modo 3 (0+3+4+5) sumador A,B,C"
  # "Modo 3 (2+3+4+5) sumador A,B,C"
  # "Modo 4 (1+2+3+4) sumador A,B,C"
  # "Modo 4 (0+3+4+5) sumador A,B,C"
  # "Modo 4 (2+3+4+5) sumador A,B,C"
  # "Modo 4 (1+2+3+4) sumador A,B,C"
  # "Modo 3 (3+4+5) sumador A,B,C"
  # "Modo 3 (2+3+4) sumador A,B,C"
  # "Modo 3 (1+2+3) sumador A,B,C"
  # "Modo 3 (3+4+5) sumador A,B,C"
  # "Modo 3 (2+3+4) sumador A,B,C"
  # "Modo 3 (1+2+3) sumador A,B,C"
  n1 = Unbundle By Name("Config Test IN") -> ("Config Test"=w5:T4)
  n2 = Index Array(array=w5, index="Vasic") -> (element=w4:T5)
  n3 = Unbundle By Name(w4) -> ("Test Rate Scan Adders?"=w1:bool)
  n4 = case shown="True" w1 {
    tunnel: "Text In" -> [w8 w53]
    tunnel: [w8 w49] -> w6
    tunnel: "Config Test IN" -> [_ w32]
    tunnel: "Vasic" -> [_ w31]
    frame False {
    }
    frame True {
      # "No conocemos el valor\nexacto de la entrada cuando sumamos\nya que es en el interior del asic\nasi que lo aproximamos con\nel valor theorico que deberia ser"
      n5 = Unbundle By Name(w32) -> ("CONFIG GEN"=w11:T12[], "Config Test"=w37:T4, "Result"=w12:T6)
      n6 = Index Array(array=w37, index=w31) -> (element=w30:T5)
      n7 = Unbundle By Name(w30) -> ("Limits Rate Scan adders.High"=w43:dbl[], "Limits Rate Scan adders.Low"=w42:dbl[], "Vin Rate Adders"=w14:i32[])
      n8 = Index Array(array=w12, index=w31) -> (element=w52:T7)
      n9 = Unbundle By Name(w30) -> ("Test offset analog?"=w28:bool, "Vasic"=w29:dbl)
      n10 = Unbundle By Name(w52) -> ("Test Rate Scan adders.Rate Scan Adders OK"=w48:bool, "Test Rate Scan adders.Volt HLTH"=w19:dbl[][][], "Test Rate Scan adders.DAC TH0,TH1,TH2"=w51:u16[][][], "Test Rate Scan adders.Add HLTH OK"=w46:bool[][][], "Test Rate Scan adders.Volt LLTH"=w18:dbl[][][], "Test Rate Scan adders.DAC TH3,TH4,TH5"=w50:u16[][][], "Test Rate Scan adders.Add LLTH 2 OK"=w45:bool[][][], "Test Rate Scan adders.OFFSET HLTH"=w21:dbl[][], "Test Rate Scan adders.OFFSET LLTH"=w20:dbl[][], "Test Rate Scan adders.Real Voltage"=w9:dbl[])
      n11 = Increment(x=w31) -> (x+1=w25:i32)
      n12 = for {
        tunnel: w14 -> [w104] mode=indexing
        tunnel: w11 -> [w107]
        tunnel: [w106] -> w10 mode=indexing
        n13 = Index Array(array=w107, index=w104) -> (element=w105:T12)
        n14 = Unbundle By Name(w105) -> ("Vasic Theorical"=w106:dbl)
      }
      n15 = Format Into String(format string="%d.5# RATE SCAN ADDERS TEST (V SUPPLY ASIC: %.3g) " ("Secction"), w25, w29) -> (resulting string=w34:string)  [unwired: 2 in, 1 out]
      n16 = disable-structure shown="Enabled" {
        disable-tunnel: w43 -> [w58 w89]
        disable-tunnel: w42 -> [w57 w88]
        disable-tunnel: [w56 w87] -> w41
        disable-tunnel: [w55 w86] -> w40
        disable-tunnel: w14 -> [w54 w90]
        frame Disabled {
          n17 = for {
            tunnel: w54 -> [w85] mode=indexing
            tunnel: w57 -> [w67]
            tunnel: w58 -> [w68]
            tunnel: [w60] -> w56 mode=indexing
            tunnel: [w59] -> w55 mode=indexing
            w72 = 4 ("x")
            w77 = 3 ("x")
            w82 = 2 ("x")
            # "numero\nde\nsumadores\n2, 3, 4"
            n18 = Increment(x=w85) -> (x+1=w69:i32)
            n19 = Multiply(x=w82, y=w69) -> (x*y=w84:i32)
            n20 = Multiply(x=w77, y=w69) -> (x*y=w75:i32)
            n21 = Multiply(x=w72, y=w69) -> (x*y=w74:i32)
            n22 = Multiply(x=w82, y=w69) -> (x*y=w83:i32)
            n23 = Multiply(x=w77, y=w69) -> (x*y=w76:i32)
            n24 = Multiply(x=w72, y=w69) -> (x*y=w73:i32)
            n25 = Decrement(x=w84) -> (x-1=w81:i32)
            n26 = Decrement(x=w75) -> (x-1=w78:i32)
            n27 = Decrement(x=w74) -> (x-1=w71:i32)
            n28 = Decrement(x=w83) -> (x-1=w80:i32)
            n29 = Decrement(x=w76) -> (x-1=w79:i32)
            n30 = Decrement(x=w73) -> (x-1=w70:i32)
            n31 = Index Array(array=w68, index=w81) -> (element=w63:dbl)
            n32 = Index Array(array=w68, index=w78) -> (element=w62:dbl)
            n33 = Index Array(array=w68, index=w71) -> (element=w61:dbl)
            n34 = Index Array(array=w67, index=w80) -> (element=w66:dbl)
            n35 = Index Array(array=w67, index=w79) -> (element=w65:dbl)
            n36 = Index Array(array=w67, index=w70) -> (element=w64:dbl)
            n37 = Build Array(w63, w62, w61) -> (w60:dbl[])
            n38 = Build Array(w66, w65, w64) -> (w59:dbl[])
          }
        }
        frame Enabled {
          n39 = for {
            tunnel: w89 -> [w103]
            tunnel: w88 -> [w102]
            tunnel: w90 -> [w101] mode=indexing
            tunnel: [w98] -> w87 mode=indexing
            tunnel: [w97] -> w86 mode=indexing
            n40 = Multiply(x=w101, y=3) -> (x*y=w99:i32)
            n41 = Index Array(array=w103, index #1=w99) -> (element #1=w96:dbl, element #2=w92:dbl, element #3=w91:dbl)  [unwired: 2 in]
            n42 = Index Array(array=w102, index #1=w99) -> (element #1=w95:dbl, element #2=w94:dbl, element #3=w93:dbl)  [unwired: 2 in]
            n43 = Build Array(w95, w94, w93) -> (w97:dbl[])
            n44 = Build Array(w96, w92, w91) -> (w98:dbl[])
          }
        }
      }
      n45 = call "REPORT.Create line.vi"("Secction"=w34, "Char"="-", "Text In"=w53) -> ("Text Out"=w38:string)  [unwired: 8 in]
      n46 = call "REPEORT.CAMBIO LINEA.vi"("Text Out"=w38) -> ("String"=w35:string)  [unwired: 8 in]
      n47 = call "REPORT.BIN TO STRING.vi"("Resultado test"=w48) -> ("OK, Fault"=w33:string)  [unwired: 14 in]
      n48 = for {
        tunnel: w21 -> [w112] mode=indexing
        tunnel: w20 -> [w111] mode=indexing
        tunnel: [w108] -> w22 mode=indexing
        n49 = for {
          tunnel: w112 -> [w116] mode=indexing
          tunnel: w111 -> [w115] mode=indexing
          tunnel: [w114] -> w110 mode=indexing
          tunnel: [w113] -> w109 mode=indexing
          n50 = Format Value(format string="%,;%1.4f", value (0)=w115) -> (output string=w113:string)  [unwired: 1 in]
          n51 = Format Value(format string="%,;%1.4f", value (0)=w116) -> (output string=w114:string)  [unwired: 1 in]
        }
        n52 = Build Array (concatenate)(w110, w109) -> (w108:string[])
      }
      n53 = Format Into String(format string="[%d.5.1# FINAL RESULT RATE SCAN ADDERS]\nRATE SCAN ADDERS TEST\\t%s" ("string"), initial string=w35, w25, w33) -> (resulting string=w39:string)  [unwired: 1 in, 1 out]
      n54 = call "REPEORT.CAMBIO LINEA.vi"("Text Out"=w39) -> ("String"=w24:string)  [unwired: 8 in]
      n55 = call "cruce por cero adders.vi"("Vin Asic Real"=w9, "Volt LLTH"=w18, "Volt HLTH"=w19) -> ("Volt LLTH Corregido"=w16:dbl[][][], "Volt HLTH Corregido"=w17:dbl[][][])  [unwired: 5 in, 2 out]
      n56 = Format Into String(format string="[%d.5.1# VALUES OFFSET RATE SCAN ADDERS ASIC]" ("Secction"), w25) -> (resulting string=w27:string)  [unwired: 2 in, 1 out]
      n57 = call "REPORT.Create Table.vi"("Secction"=w27, "Row Headers"=string[] ["MODE 2 (2+4)", "MODE 2 (3+4)", "MODE 2 (4+5)", "MODE 3 (2+3+4)", "MODE 3 (3+4+5)", "MODE 3 (4+5+6)", "MODE 4 (2+3+4+5)", "MODE 4 (3+4+5+6)", "MODE 4 (1+4+5+6)"] ("Column Headers"), "Column Headers"=string[] ["ADD A OUT 0", "ADD B OUT 0", "ADD C OUT 0", "ADD A OUT 1", "ADD B OUT 1", "ADD C OUT 1"], "Text 2d"=w22, "Text In"=w24) -> ("Text Out"=w23:string)  [unwired: 3 in, 1 out]
      n58 = for {
        tunnel: w19 -> [w136] mode=indexing
        tunnel: w51 -> [w200] mode=indexing
        tunnel: w18 -> [w143] mode=indexing
        tunnel: w50 -> [w199] mode=indexing
        shift-right: [w167] -> w49
        shift-left: w23 -> [w186]
        tunnel: w11 -> [w123]
        tunnel: w14 -> [w121] mode=indexing
        tunnel: w46 -> [w132] mode=indexing
        tunnel: w45 -> [w131] mode=indexing
        tunnel: w41 -> [w171]
        tunnel: w40 -> [w169]
        tunnel: w25 -> [w148]
        tunnel: w29 -> [w146]
        tunnel: w28 -> [_]
        tunnel: w17 -> [w128] mode=indexing
        tunnel: w16 -> [w127] mode=indexing
        tunnel: w10 -> [_] mode=indexing
        tunnel: w9 -> [w119] mode=indexing
        i -> [w159]
        w137 = dbl[] [2.0, 2.0, 2.0, 3.0, 3.0, 3.0, 4.0, 4.0, 4.0]
        w145 = string[] ["MODE 2 (2+4)", "MODE 2 (3+4)", "MODE 2 (4+5)", "MODE 3 (2+3+4)", "MODE 3 (3+4+5)", "MODE 3 (4+5+6)", "MODE 4 (2+3+4+5)", "MODE 4 (3+4+5+6)", "MODE 4 (1+4+5+6)"] ("Column Headers")
        w144 = string[] ["ADD A OUT 0", "ADD B OUT 0", "ADD C OUT 0", "ADD A OUT 1", "ADD B OUT 1", "ADD C OUT 1"] ("Row Headers")
        n59 = Index Array(array=w123, index=w121) -> (element=w125:T12)
        n60 = Divide(x=w127, y=w119) -> (x/y=w138:dbl[][])
        n61 = Divide(x=w128, y=w119) -> (x/y=w135:dbl[][])
        n62 = Transpose 2D Array(2D array=w135) -> (transposed array=w142:dbl[][])
        n63 = Transpose 2D Array(2D array=w138) -> (transposed array=w139:dbl[][])
        n64 = Index Array(array=w123, index=w121) -> (element=w122:T12)
        n65 = Unbundle By Name(w125) -> ("Vasic Theorical"=w124:dbl)
        n66 = for {
          tunnel: w142 -> [w244] mode=indexing
          tunnel: w137 -> [w243]
          tunnel: [w242] -> w141 mode=indexing
          n67 = Divide(x=w244, y=w243) -> (x/y=w242:dbl[])
        }
        n68 = Array Size(array=w132) -> (size(s)=w181:i32[])
        n69 = for {
          tunnel: w139 -> [w241] mode=indexing
          tunnel: [w240] -> w140 mode=indexing
          tunnel: w137 -> [w239]
          n70 = Divide(x=w241, y=w239) -> (x/y=w240:dbl[])
        }
        n71 = Unbundle By Name(w122) -> ("Amplitude"=w120:dbl, "Width Time"=w174:dbl, "Frequency"=w197:dbl)
        n72 = Index Array(array=w171, index (row)=w159) -> (element=w170:dbl[])  [unwired: 1 in]
        n73 = Index Array(array=w169, index (row)=w159) -> (element=w168:dbl[])  [unwired: 1 in]
        n74 = Index Array(array=w181, index #1=0 ("index")) -> (element #1=w179:i32, element #2=w178:i32)  [unwired: 1 in]
        n75 = Transpose 2D Array(2D array=w141) -> (transposed array=w133:dbl[][])
        n76 = Transpose 2D Array(2D array=w140) -> (transposed array=w134:dbl[][])
        n77 = Add(x=3, y=w159) -> (x+y=w147:i32)
        n78 = for {
          tunnel: [w247] -> w172 mode=indexing
          tunnel: w170 -> [w246] mode=indexing
          tunnel: w168 -> [w245] mode=indexing
          n79 = Format Value(format string="%,;%1.4f", value (0)=w245) -> (output string=w248:string)  [unwired: 1 in]
          n80 = Format Value(format string="%,;%1.4f", value (0)=w246) -> (output string=w249:string)  [unwired: 1 in]
          n81 = Build Array(w249, w248) -> (w247:string[])
        }
        n82 = for {
          tunnel: w136 -> [w260] mode=indexing
          tunnel: w200 -> [w259] mode=indexing
          tunnel: w143 -> [w258] mode=indexing
          tunnel: w199 -> [w257] mode=indexing
          tunnel: [w254] -> w189 mode=indexing
          tunnel: w132 -> [w253] mode=indexing
          tunnel: w131 -> [w252] mode=indexing
          n83 = for {
            tunnel: w260 -> [w298] mode=indexing
            tunnel: w259 -> [w265] mode=indexing
            tunnel: w258 -> [w297] mode=indexing
            tunnel: w257 -> [w275] mode=indexing
            tunnel: [w289] -> w256 mode=indexing
            tunnel: [w284] -> w255 mode=indexing
            tunnel: w253 -> [w262] mode=indexing
            tunnel: w252 -> [w261] mode=indexing
            w263 = " (%02d.%01d)" ("format string")
            w295 = "%,;%1.4f" ("format string")
            n84 = Format Value(format string=w295, value (0)=w298) -> (output string=w296:string)  [unwired: 1 in]
            n85 = Format Value(format string=w295, value (0)=w297) -> (output string=w294:string)  [unwired: 1 in]
            n86 = Number To Boolean Array(number=w265) -> (Boolean array=w266:bool[])
            n87 = Number To Boolean Array(number=w275) -> (Boolean array=w283:bool[])
            n88 = Split 1D Array(array=w266, index=2) -> (first subarray=w270:bool[], second subarray=w269:bool[])
            n89 = Split 1D Array(array=w283, index=2) -> (first subarray=w279:bool[], second subarray=w280:bool[])
            n90 = Index Array(array=w270) -> (element #1=w271:bool, element #2=w273:bool)  [unwired: 2 in]
            n91 = Boolean Array To Number(Boolean array=w269) -> (number=w268:u32)
            n92 = Index Array(array=w279) -> (element #1=w278:bool, element #2=w276:bool)  [unwired: 2 in]
            n93 = Boolean Array To Number(Boolean array=w280) -> (number=w281:u32)
            n94 = Boolean To (0,1)(Boolean=w273) -> (0, 1=w272:i16)
            n95 = Boolean To (0,1)(Boolean=w271) -> ()  [unwired: 1 out]
            n96 = Boolean To (0,1)(Boolean=w276) -> (0, 1=w277:i16)
            n97 = Boolean To (0,1)(Boolean=w278) -> ()  [unwired: 1 out]
            n98 = Format Into String(format string=w263, w268, w272) -> (resulting string=w264:string)  [unwired: 2 in, 1 out]
            n99 = Format Into String(format string=w263, w281, w277) -> (resulting string=w274:string)  [unwired: 2 in, 1 out]
            n100 = Select(t="", s=w262, f="*") -> (s? t:f=w291:string)
            n101 = Select(t="", s=w261, f="*") -> (s? t:f=w285:string)
            n102 = Concatenate Strings(w296, w264) -> (w290:string)
            n103 = Concatenate Strings(w294, w274) -> (w286:string)
            n104 = Concatenate Strings(w290, w291) -> (w289:string)
            n105 = Concatenate Strings(w286, w285) -> (w284:string)
          }
          n106 = Build Array (concatenate)(w256, w255) -> (w254:string[])
        }
        n107 = for {
          tunnel: w132 -> [w209] mode=indexing
          tunnel: w131 -> [w208] mode=indexing
          tunnel: [w205] -> w130 mode=indexing
          tunnel: w128 -> [w204] mode=indexing
          tunnel: w133 -> [w202] mode=indexing
          tunnel: w127 -> [w203] mode=indexing
          tunnel: w134 -> [w201] mode=indexing
          n108 = for {
            tunnel: w209 -> [w212] mode=indexing
            tunnel: w208 -> [w211] mode=indexing
            tunnel: [w218] -> w207 mode=indexing
            tunnel: [w217] -> w206 mode=indexing
            tunnel: w204 -> [w216] mode=indexing
            tunnel: w202 -> [w215] mode=indexing
            tunnel: w203 -> [w214] mode=indexing
            tunnel: w201 -> [w213] mode=indexing
            w210 = " (%,;%1.4f)" ("format string")
            w229 = "%,;%1.4f" ("format string")
            n109 = Format Value(format string=w210, value (0)=w215) -> (output string=w230:string)  [unwired: 1 in]
            n110 = Format Value(format string=w229, value (0)=w214) -> (output string=w227:string)  [unwired: 1 in]
            n111 = Format Value(format string=w210, value (0)=w213) -> (output string=w231:string)  [unwired: 1 in]
            n112 = Format Value(format string=w229, value (0)=w216) -> (output string=w228:string)  [unwired: 1 in]
            n113 = Concatenate Strings(w227, w231) -> (w220:string)
            n114 = Concatenate Strings(w228, w230) -> (w223:string)
            n115 = Select(t="", s=w212, f="*") -> (s? t:f=w224:string)
            n116 = Select(t="", s=w211, f="*") -> (s? t:f=w219:string)
            n117 = Concatenate Strings(w223, w224) -> (w218:string)
            n118 = Concatenate Strings(w220, w219) -> (w217:string)
          }
          n119 = Build Array (concatenate)(w207, w206) -> (w205:string[])
        }
        n120 = Initialize Array(TRUE, w179, w178) -> (w184:bool[][])
        n121 = Equal?(x=w132, y=w184) -> (x = y?=w183:bool)
        n122 = Equal?(x=w131, y=w184) -> (x = y?=w182:bool)
        n123 = Format Into String(format string="[%d.5.%d.1# VOLTAGE INPUT ASIC]\nV Theorical\\t%,;%1.4f\nV Real\\t%,;%1.4f" ("Secction"), initial string=w186, w148, w147, w124, w119) -> (resulting string=w156:string)  [unwired: 1 in, 1 out]
        n124 = And(x=w183, y=w182) -> (x .and. y?=w177:bool)
        n125 = call "REPEORT.CAMBIO LINEA.vi"("Text Out"=w156) -> ("String"=w155:string)  [unwired: 8 in]
        n126 = call "REPORT.BIN TO STRING.vi"("Resultado test"=w177) -> ("OK, Fault"=w157:string)  [unwired: 14 in]
        n127 = Format Value(format string="%,;%1.4f", value (0)=w120) -> (output string=w196:string)  [unwired: 1 in]
        n128 = Format Value(format string="%,;%^#_6e", value (0)=w174) -> (output string=w175:string)  [unwired: 1 in]
        n129 = Format Value(format string="%,;%^#_6e", value (0)=w197) -> (output string=w195:string)  [unwired: 1 in]
        n130 = Format Into String(format string="[%d.5.%d.2# RESULT OF TEST RATE SCAN ADDERS (V IN)]\nRATE SCAN ADDERS VIN\\t%s" ("string"), initial string=w155, w148, w147, w157) -> (resulting string=w154:string)  [unwired: 1 in, 1 out]
        n131 = call "REPEORT.CAMBIO LINEA.vi"("Text Out"=w154) -> ("String"=w153:string)  [unwired: 8 in]
        n132 = Build Array(w196, w175, w195) -> (w192:string[])
        n133 = Format Into String(format string="%d.5.%d.3# LIMITS COMPARATION RATE SCAN ADDERS" ("Secction"), w148, w147) -> (resulting string=w163:string)  [unwired: 2 in, 1 out]
        n134 = Build Array(w192) -> (w191:string[][])
        n135 = call "REPORT.Create Table.vi"("Secction"=w163, "Row Headers"=string[] ["MODE 2", "MODE 3", "MODE 4"], "Column Headers"=string[] ["UPPER", "LOWER"], "Text 2d"=w172, "Text In"=w153) -> ("Text Out"=w188:string)  [unwired: 3 in, 1 out]
        n136 = Format Into String(format string="%d.5.%d.4# VGA PARAMETERS RATE SCAN  ADDERS" ("string"), w148, w147) -> (resulting string=w162:string)  [unwired: 2 in, 1 out]
        n137 = call "REPORT.Create Table.vi"("Secction"=w162, "Column Headers"=string[] ["Amplitude (Volt)", "PULSE WIDTH (Seg)", "FRECUENCY (Hz)"], "Text 2d"=w191, "Text In"=w188) -> ("Text Out"=w190:string)  [unwired: 4 in, 1 out]
        n138 = Format Into String(format string="%d.5.%d.5# VALUES RATE SCAN ADDERS ASIC (%.3g@%1.4f) " ("Secction"), w148, w147, w146, w124) -> (resulting string=w160:string)  [unwired: 2 in, 1 out]
        n139 = call "REPORT.Create Table.vi"("Secction"=w160, "Row Headers"=w145, "Column Headers"=w144, "Text 2d"=w189, "Text In"=w190) -> ("Text Out"=w150:string)  [unwired: 3 in, 1 out]
        n140 = Format Into String(format string="%d.5.%d.6# VALUES RATE SCAN ADDERS ASIC RECTIFIED (%.3g@%1.4f) " ("Secction"), w148, w147, w146, w124) -> (resulting string=w151:string)  [unwired: 2 in, 1 out]
        n141 = case shown="True" TRUE {
          tunnel: w151 -> [_ w238]
          tunnel: w150 -> [w232 w237]
          tunnel: [w232 w236] -> w149
          tunnel: w145 -> [_ w235]
          tunnel: w144 -> [_ w234]
          tunnel: w130 -> [_ w233]
          frame False {
          }
          frame True {
            n142 = call "REPORT.Create Table.vi"("Secction"=w238, "Row Headers"=w235, "Column Headers"=w234, "Text 2d"=w233, "Text In"=w237) -> ("Text Out"=w236:string)  [unwired: 3 in, 1 out]
          }
        }
        n143 = call "REPEORT.CAMBIO LINEA.vi"("Text Out"=w149) -> ("String"=w167:string)  [unwired: 8 in]
      }
    }
  }
  "Text Out" <- w6
